vi "pb_init.vi"(8 "error in (no error)":errorcluster, 11 "path in":path=path "C:/SpinCore/SpinAPI/lib/spinapi64.dll") -> (0 "error out":errorcluster, 3 "path out":path)   [LabVIEW 2018]
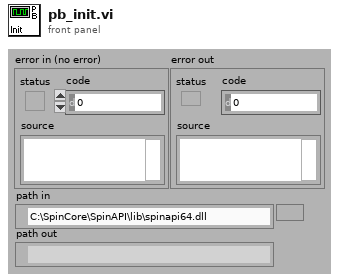
[diagram p1: front panel]
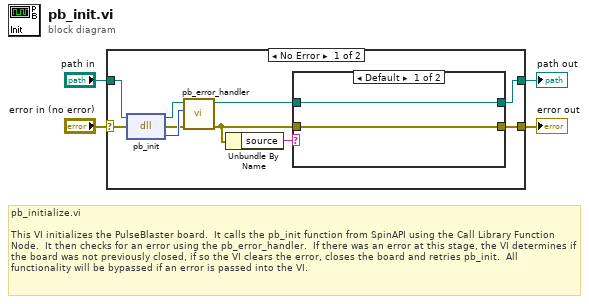
[diagram p0: block diagram]
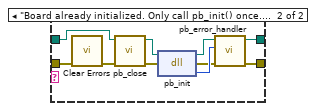
[diagram p2: hidden frame]
diagram:
  # "pb_initialize.vi\n\nThis VI initializes the PulseBlaster board.  It calls the pb_init function from SpinAPI using the Call Library Function Node.  It then checks for an error using the pb_error_handler.  If there was an error at this stage, the VI determines if the board was not previously closed, if so the VI clears the error, closes the board and retries pb_init.  All functionality will be bypassed if an error is passed into the VI."
  n1 = case shown="No Error" "error in (no error)" {
    selector: "error in (no error)" -> [w13 w28]
    tunnel: [w7 w28] -> w4
    tunnel: [w6 w27] -> w2
    tunnel: "path in" -> [w5 w27]
    frame No Error {
      n2 = dll-call lib="C:/SpinCore/SpinAPI/lib/spinapi64.dll" fn="pb_init"(path in=w5, error in=w13) -> (path out=w12:path, error out=w11:errorcluster, "return type"=w14:i32)  [unwired: 1 in]
      n3 = call "pb_error_handler.vi"("error in (no error)"=w11, "return code"=w14, "path in"=w12) -> ("error out"=w9:errorcluster, "path out"=w8:path)  [unwired: 7 out]
      n4 = Unbundle By Name(w9) -> ("source"=w10:string)
      n5 = case shown="Default" w10 {
        tunnel: [w15 w25] -> w6
        tunnel: w9 -> [w16 w24]
        tunnel: w8 -> [w15 w22]
        tunnel: [w16 w17] -> w7
        frame Default {
        }
        frame "Board already initialized. Only call pb_init() once." {
          n6 = call <vilib>:"Clear Errors.vi"("error in (no error)"=w24) -> ("error out"=w23:errorcluster)  [unwired: 1 in, 5 out]
          n7 = call "pb_close.vi"("error in (no error)"=w23, "path in"=w22) -> ("error out"=w20:errorcluster, "path out"=w21:path)  [unwired: 8 out]
          n8 = dll-call lib="C:/Program Files/SpinCore/SpinAPI/dll/spinapi.dll" fn="pb_init"(path in=w21, error in=w20) -> (path out=w19:path, error out=w18:errorcluster, "return type"=w26:i32)  [unwired: 1 in]
          n9 = call "pb_error_handler.vi"("error in (no error)"=w18, "return code"=w26, "path in"=w19) -> ("error out"=w17:errorcluster, "path out"=w25:path)  [unwired: 7 out]
        }
      }
    }
    frame Error {
    }
  }
  "error out" <- w4
  "path out" <- w2
